vi "Read Helm Rate (Hz) Actor.vi"(8 "error in (no error)":errorcluster, 11 "RDS Helm Actor in":refnum<class "RDS Helm Actor.lvclass">) -> (0 "error out":errorcluster, 2 "Helm Rate (Hz)":dbl, 3 "RDS Helm Actor out":refnum<class "RDS Helm Actor.lvclass">)   [LabVIEW 2015, in "RDS Helm Actor.lvlib" / "RDS Helm Actor.lvclass"]
uses:
  RDS Helm Actor.lvclass
  RDS Helm Actor.lvclass/RDS Helm Actor.ctl
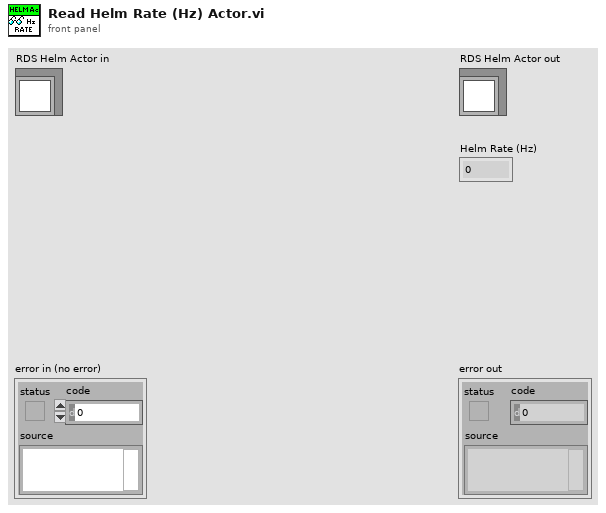
[diagram p1: front panel]
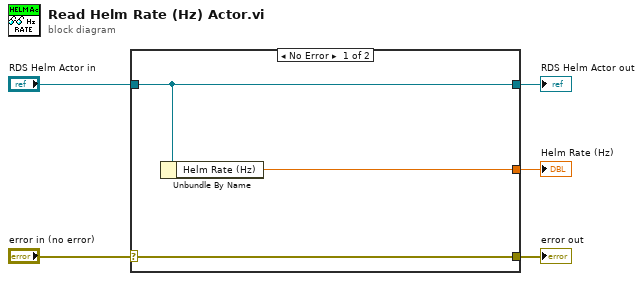
[diagram p0: block diagram]
diagram:
  n1 = case shown="No Error" "error in (no error)" {
    selector: "error in (no error)" -> [w8 w9]
    tunnel: [w8 w9] -> w4
    tunnel: [w7 w10] -> w2
    tunnel: "RDS Helm Actor in" -> [w7 w10]
    tunnel: [w6 _] -> w1
    frame No Error {
      n2 = Unbundle By Name(w7) -> ("Helm Rate (Hz)"=w6:sgl)
    }
    frame Error {
    }
  }
  "error out" <- w4
  "RDS Helm Actor out" <- w2
  "Helm Rate (Hz)" <- w1
